vi "Digitizer_Mode_Init.vi"(8 "error in":errorcluster, 11 "Channel Parameters In":T1) -> (0 "error out":errorcluster, 1 "Waveforms Out (Empty)":T2(array[cluster]), 3 "dup Channel Parameters Out":T1)   [LabVIEW 2010]
uses:
  Typedef-Channel Parameters.ctl
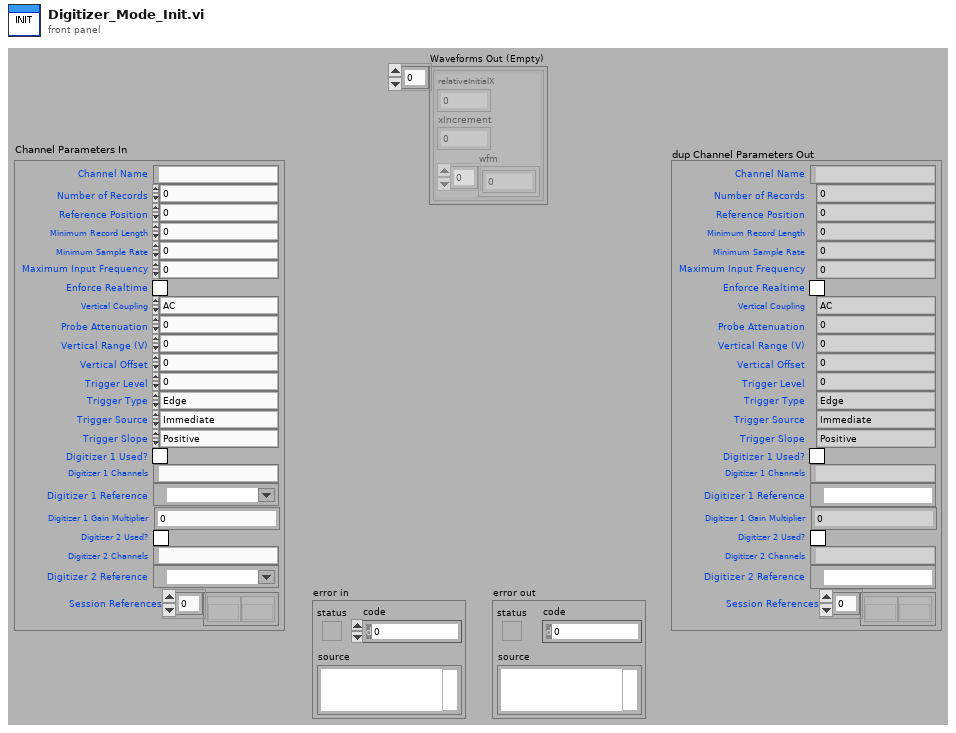
[diagram p1: front panel]
types:
  T1 = typedef "Typedef-Channel Parameters.ctl" = cluster{"Channel Name":string, "Number of Records":i32, "Reference Position":dbl, "Minimum Record Length":i32, "Minimum Sample Rate":dbl, "Maximum Input Frequency":dbl, "Enforce Realtime":bool, "Vertical Coupling":enum16{"AC", "DC", "Ground"}, "Probe Attenuation":dbl, "Vertical Range (V)":dbl, "Vertical Offset":dbl, "Trigger Level":dbl, "Trigger Type":enum16{"Edge", "Digital", "Immediate"}, "Trigger Source":enum16{"Immediate", "Channel 0", "Channel 1", "Channel 2", "Channel 3", "Channel 4", "Channel 5", "Channel 6", "Channel 7", "Extermal TRIG", "Software Trigger", "RTSI 0", "RTSI 1", "RTSI 2", "RTSI 3", "RTSI 4", "RTSI 5", "RTSI 6", "PF 0", "PF 1", "PF 2", "PXI Star Trigger"}, "Trigger Slope":enum16{"Positive", "Negative"}, "Digitizer 1 Used?":bool, "Digitizer 1 Channels":string, "Digitizer 1 Reference":refnum<k15>, "Digitizer 1 Gain Multiplier":dbl, "Digitizer 2 Used?":bool, "Digitizer 2 Channels":string, "Digitizer 2 Reference":refnum<k15>, "Session References":refnum<k20>[]}
  T2 = cluster{"relativeInitialX":dbl, "xIncrement":dbl, "wfm":dbl[]}[]
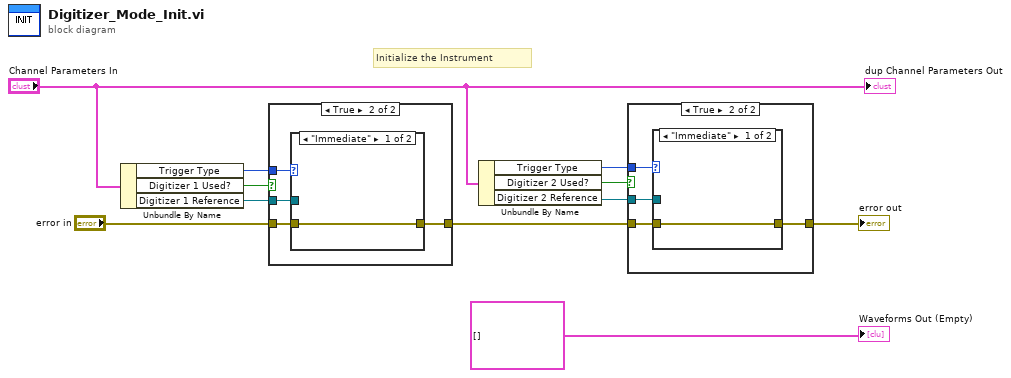
[diagram p0: block diagram]
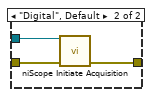
[diagram p3: hidden frame]
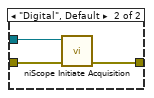
[diagram p5: hidden frame]
diagram:
  # "Initialize the Instrument"
  n1 = Unbundle By Name("Channel Parameters In") -> ("Trigger Type"=w9:enum16{"Edge", "Digital", "Immediate"}, "Digitizer 1 Used?"=w3:bool, "Digitizer 1 Reference"=w4:refnum<k15>)
  n2 = case shown="True" w3 {
    tunnel: "error in" -> [w12 w15]
    tunnel: w4 -> [_ w16]
    tunnel: [w12 w14] -> w1
    tunnel: w9 -> [_ w13]
    frame False {
    }
    frame True {
      n3 = case shown="\"Immediate\"" w13 {
        tunnel: w16 -> [_ w18]
        tunnel: w15 -> [w17 w19]
        tunnel: [w17 w20] -> w14
        frame "Immediate" {
        }
        frame "Digital", Default {
          n4 = call <instrlib>:"niScope Initiate Acquisition.vi"("instrument handle"=w18, "error in"=w19) -> ("error out"=w20:errorcluster)  [unwired: 12 in, 1 out]
        }
      }
    }
  }
  n5 = Unbundle By Name("Channel Parameters In") -> ("Trigger Type"=w10:enum16{"Edge", "Digital", "Immediate"}, "Digitizer 2 Used?"=w6:bool, "Digitizer 2 Reference"=w7:refnum<k15>)
  n6 = case shown="True" w6 {
    tunnel: w1 -> [w21 w23]
    tunnel: w7 -> [_ w24]
    tunnel: [w21 w25] -> w2
    tunnel: w10 -> [_ w22]
    frame False {
    }
    frame True {
      n7 = case shown="\"Immediate\"" w22 {
        tunnel: w24 -> [_ w27]
        tunnel: w23 -> [w26 w28]
        tunnel: [w26 w29] -> w25
        frame "Immediate" {
        }
        frame "Digital", Default {
          n8 = call <instrlib>:"niScope Initiate Acquisition.vi"("instrument handle"=w27, "error in"=w28) -> ("error out"=w29:errorcluster)  [unwired: 12 in, 1 out]
        }
      }
    }
  }
  "error out" <- w2
  "Waveforms Out (Empty)" <- T2 []
  "dup Channel Parameters Out" <- "Channel Parameters In"
